vi "unreserve resource.vi"(8 "error in (no error)":errorcluster, 9 "Name in Bitfile":string, 10 "Server Ref in":T1 format="%.0x", 11 "Item Ref in":T1 format="%.0x") -> (0 "error out":errorcluster, 3 "Item Ref out":T1 format="%.0x")   [LabVIEW 2016, in "RM.Client.lvlib"]
uses:
  RM.Client.lvlib
  <vilib>/NI Veristand/Custom Device API/Custom Device Item Ref.ctl
  Server/RM.Server.lvlib
  <vilib>/NI VeriStand/Custom Device API/Custom Device API.lvlib
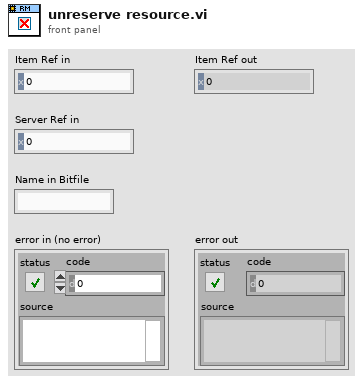
[diagram p1: front panel]
types:
  T1 = typedef "Custom Device API.lvlib/Custom Device Item Ref.ctl" = u64
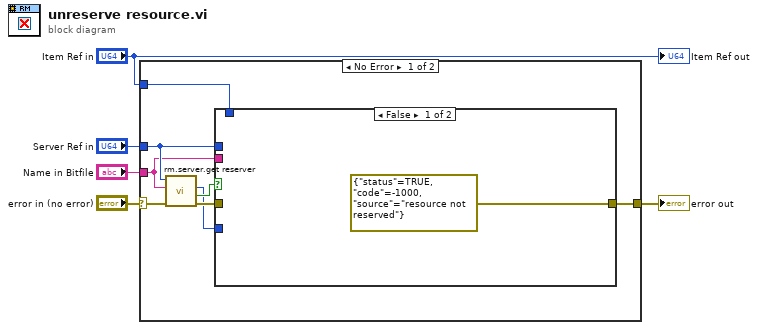
[diagram p0: block diagram]
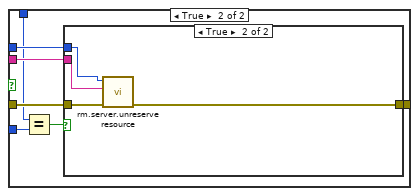
[diagram p2: hidden frame]
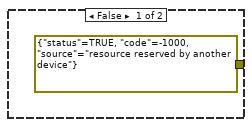
[diagram p3: hidden frame]
diagram:
  n1 = case shown="No Error" "error in (no error)" {
    selector: "error in (no error)" -> [w10 w27]
    tunnel: [w13 w27] -> w4
    tunnel: "Item Ref in" -> [w6 _]
    tunnel: "Server Ref in" -> [w12 _]
    tunnel: "Name in Bitfile" -> [w11 _]
    frame No Error {
      n2 = call "rm.server.get reserver.vi"("error in (no error)"=w10, "Name in Bitfile"=w11, "Item Ref in"=w12) -> ("error out"=w9:errorcluster, "found?"=w8:bool, "Reserver Node Ref"=w7:T1)  [unwired: 5 in, 1 out]
      n3 = case shown="False" w8 {
        tunnel: [errorcluster {"status"=TRUE, "code"=-1000, "source"="resource not reserved"} ("error out") w21] -> w13
        tunnel: w12 -> [_ w20]
        tunnel: w11 -> [_ w19]
        tunnel: w9 -> [_ w18]
        tunnel: w7 -> [_ w16]
        tunnel: w6 -> [_ w15]
        frame False {
        }
        frame True {
          n4 = Equal?(x=w15, y=w16) -> (x = y?=w17:bool)
          n5 = case shown="True" w17 {
            tunnel: [errorcluster {"status"=TRUE, "code"=-1000, "source"="resource reserved by another device"} ("error out") w26] -> w21
            tunnel: w20 -> [_ w25]
            tunnel: w19 -> [_ w24]
            tunnel: w18 -> [_ w23]
            frame False {
            }
            frame True {
              n6 = call "rm.server.unreserve resource.vi"("error in (no error)"=w23, "Name in bitfile"=w24, "Item Ref in"=w25) -> ("error out"=w26:errorcluster)  [unwired: 6 in, 2 out]
            }
          }
        }
      }
    }
    frame Error {
    }
  }
  "error out" <- w4
  "Item Ref out" <- "Item Ref in"
